vi "__init__.vi"(4 "Label":T2, 6 "operation":T1=enum."add", 7 "Previous":variant, 8 "error in (no error)":errorcluster, 9 "Other":variant, 10 "data":T3, 11 "Value in":refnum<class "Value.lvclass">) -> (0 "error out":errorcluster, 3 "Value out":refnum<class "Value.lvclass">)   [LabVIEW 2023, in "LabGRAD.lvlib" / "Value.lvclass"]
uses:
  Value.lvclass
  UiObjects/numeric value control.ctl
  UiObjects/string control.ctl
  operation.ctl
  Value.lvclass/Value.ctl
  UiObjects/UiObjects.lvclass
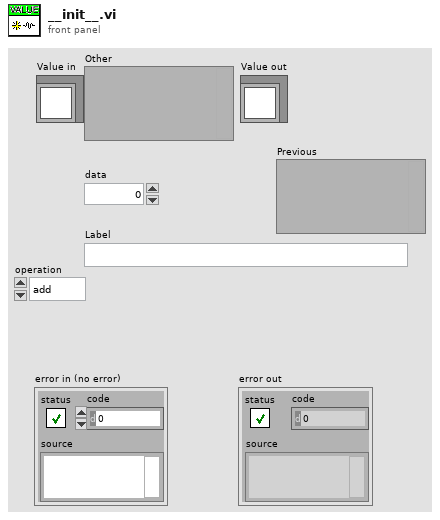
[diagram p1: front panel]
types:
  T1 = typedef "LabGRAD.lvlib/Value.lvclass/operation.ctl" = enum16{"nop", "add", "subtract", "power", "multiply", "divide"}
  T2 = typedef "UiObjects.lvlib/UiObjects.lvclass/string control.ctl" = string
  T3 = typedef "UiObjects.lvlib/UiObjects.lvclass/numeric value control.ctl" = dbl
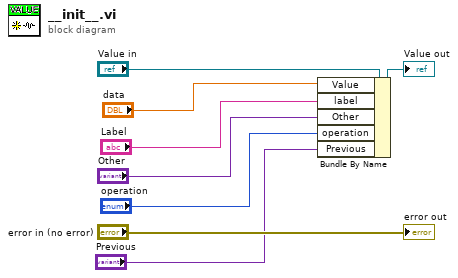
[diagram p0: block diagram]
diagram:
  n1 = Bundle By Name(cluster="Value in", "Value"="data", "label"="Label", "Other"="Other", "operation"="operation", "Previous"="Previous") -> (→"Value out":refnum<class "Value.lvclass">)
  "error out" <- "error in (no error)"
